vi "PID Structure Conversion (core).vi"(7 "PID structure":u16(ring) items=["Academic (Standard)", "Parallel", "Series"], 9 "derivative in":dbl, 10 "integral in":dbl, 11 "proportional in":dbl) -> (1 "derivative time (s)":dbl, 2 "integral time (s)":dbl, 3 "proportional":dbl)   [LabVIEW 2020, in "NI_PID_pid.lvlib"]
uses:
  <vilib>/addons/control/pid/NI_PID_pid.lvlib
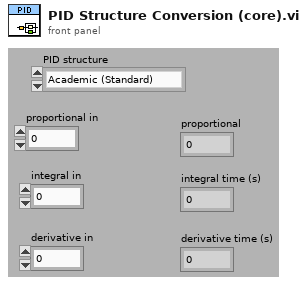
[diagram p1: front panel]
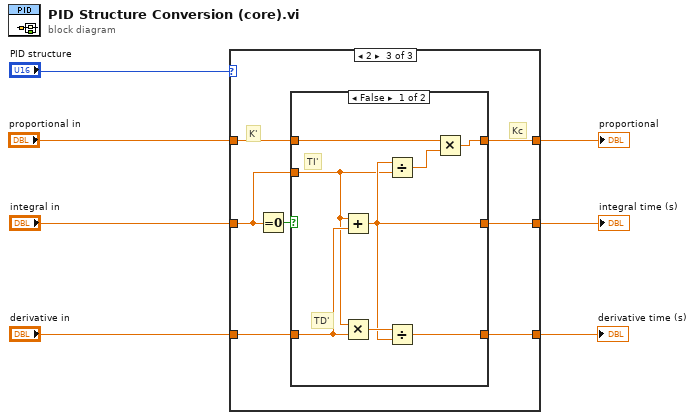
[diagram p0: block diagram]
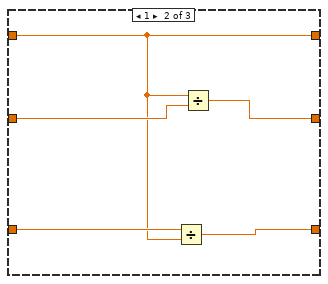
[diagram p3: hidden frame]
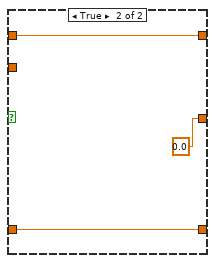
[diagram p4: hidden frame]
diagram:
  n1 = case shown="2" "PID structure" {
    tunnel: "derivative in" -> [w10 w13 w20]
    tunnel: "integral in" -> [w9 w15 w16]
    tunnel: [w10 w11 w18] -> w4
    tunnel: [w9 w14 w19] -> w5
    tunnel: [w8 w12 w21] -> w7
    tunnel: "proportional in" -> [w8 w12 w22]
    frame 0, Default {
      # "Td"
      # "Ti"
      # "Kc"
    }
    frame 1 {
      n2 = Divide(x=w13, y=w12) -> (x/y=w11:dbl)
      n3 = Divide(x=w12, y=w15) -> (x/y=w14:dbl)
    }
    frame 2 {
      # "K'"
      # "Kc"
      n4 = Equal To 0?(x=w16) -> (x = 0?=w17:bool)
      n5 = case shown="False" w17 {
        tunnel: w22 -> [w30 w33]
        tunnel: [w28 w33] -> w21
        tunnel: w20 -> [w27 w31]
        tunnel: [w25 0.0] -> w19
        tunnel: [w24 w31] -> w18
        tunnel: w16 -> [w23 _]
        frame False {
          # "TD'"
          # "TI'"
          n6 = Add(x=w23, y=w27) -> (x+y=w25:dbl)
          n7 = Multiply(x=w23, y=w27) -> (x*y=w26:dbl)
          n8 = Divide(x=w25, y=w23) -> (x/y=w29:dbl)
          n9 = Divide(x=w26, y=w25) -> (x/y=w24:dbl)
          n10 = Multiply(x=w30, y=w29) -> (x*y=w28:dbl)
        }
        frame True {
        }
      }
    }
  }
  "proportional" <- w7
  "integral time (s)" <- w5
  "derivative time (s)" <- w4
